vi "Add.vi"() -> ()   [LabVIEW 2020, in "Basic_Operations.lvlib"]
uses:
  Basic_Operations.lvlib
panel:
  out "Sum Result":dbl
  in  "B":dbl=20.0
  in  "A":dbl=10.0
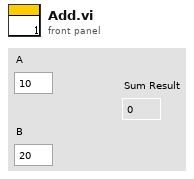
[diagram p1: front panel]
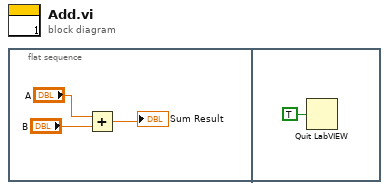
[diagram p0: block diagram]
diagram:
  n1 = flat-sequence {
    frame #0 {
      n2 = Add(x="A", y="B") -> (x+y=→"Sum Result":dbl)
    }
    frame #1 {
      n3 = Quit LabVIEW(quit? (T)=TRUE) -> ()
    }
  }
